vi "Variant_to_string_Core.vi"(11 "Value":variant) -> (3 "1D_Array_String_Setting_Name_Value":string[](array[string]))   [LabVIEW 2011]
uses:
  <vilib>/Utility/VariantDataType/VariantType.lvlib
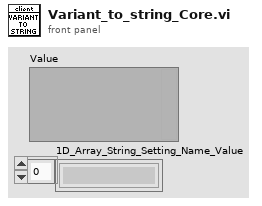
[diagram p1: front panel]
types:
  T1 = typedef "VariantType.lvlib/Type.ctl" = enum8{"Invalid Type", "Void", "I8", "I16", "I32", "I64", "U8", "U16", "U32", "U64", "Single Float", "Double Float", "Extended Float", "Single Complex", "Double Complex", "Extended Complex", "Enum U8", "Enum U16", "Enum U32", "Enum U64", "Single Float With Unit", "Double Float With Unit", "Extended Float With Unit", "Single Complex with Unit", "Double Complex with Unit", "Extended Complex with Unit", "Boolean", "String", "Path", "Picture", "Tag", "Array", "Cluster", "Variant", "LV Variant", "Waveform", "Timestamp", "Digital Waveform", "Digital Data", "ExpressData", "Refnum", "External Data", "VI", "Poly VI", "LabVIEW Class Instance", "Fixed Point"}
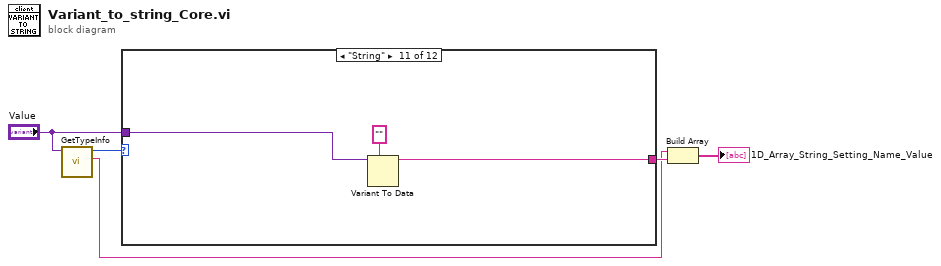
[diagram p0: block diagram]
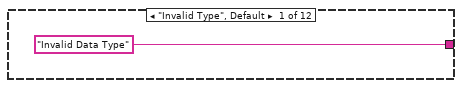
[diagram p2: hidden frame]
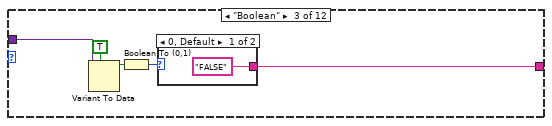
[diagram p4: hidden frame]
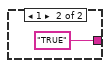
[diagram p5: hidden frame]
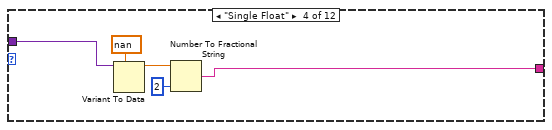
[diagram p6: hidden frame]
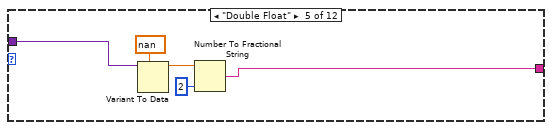
[diagram p7: hidden frame]
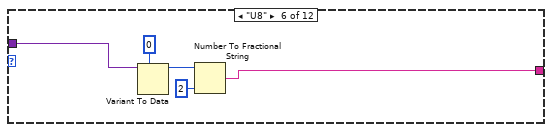
[diagram p8: hidden frame]
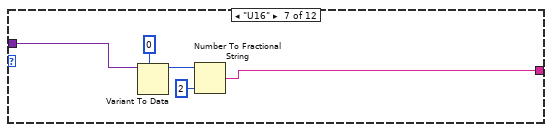
[diagram p9: hidden frame]
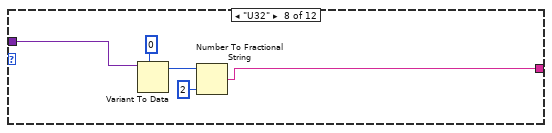
[diagram p10: hidden frame]
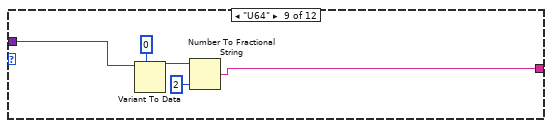
[diagram p11: hidden frame]
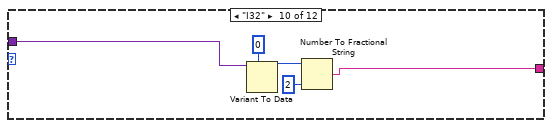
[diagram p12: hidden frame]
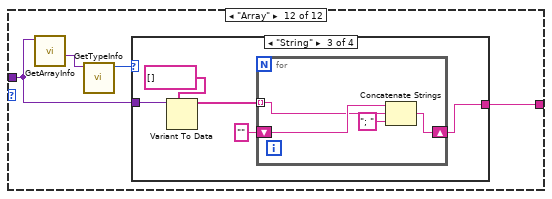
[diagram p13: hidden frame]
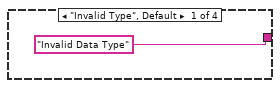
[diagram p14: hidden frame]
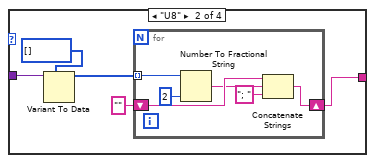
[diagram p15: hidden frame]
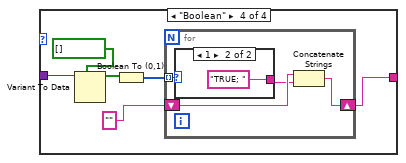
[diagram p16: hidden frame]
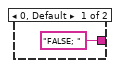
[diagram p17: hidden frame]
diagram:
  n1 = call <vilib>:"GetTypeInfo.vi"("Variant"="Value") -> ("Name"=w2:string, "Type Enum"=w4:T1)  [unwired: 6 in, 3 out]
  n2 = case shown="\"String\"" w4 {
    tunnel: "Value" -> [_ _ w7 w18 w23 w28 w33 w38 w43 w48 w51 w55]
    tunnel: ["Invalid Data Type" _ w10 w15 w20 w25 w30 w34 w39 w44 w49 w52] -> w3
    frame "Invalid Type", Default {
    }
    frame "Enum U16" {
    }
    frame "Boolean" {
      n3 = Variant To Data(type=TRUE, Variant=w7) -> (data=w8:bool)  [unwired: 1 in, 1 out]
      n4 = Boolean To (0,1)(Boolean=w8) -> (0, 1=w11:i16)
      n5 = case shown="0, Default" w11 {
        tunnel: ["FALSE" "TRUE"] -> w10
        frame 0, Default {
        }
        frame 1 {
        }
      }
    }
    frame "Single Float" {
      n6 = Variant To Data(type=sgl nan, Variant=w18) -> (data=w16:sgl)  [unwired: 1 in, 1 out]
      n7 = Number To Fractional String(number=w16, precision (6)=i16 2) -> (F-format string=w15:string)  [unwired: 2 in]
    }
    frame "Double Float" {
      n8 = Variant To Data(type=nan, Variant=w23) -> (data=w21:dbl)  [unwired: 1 in, 1 out]
      n9 = Number To Fractional String(number=w21, precision (6)=i16 2) -> (F-format string=w20:string)  [unwired: 2 in]
    }
    frame "U8" {
      n10 = Variant To Data(type=u8 0, Variant=w28) -> (data=w27:u8)  [unwired: 1 in, 1 out]
      n11 = Number To Fractional String(number=w27, precision (6)=i16 2) -> (F-format string=w25:string)  [unwired: 2 in]
    }
    frame "U16" {
      n12 = Variant To Data(type=u16 0, Variant=w33) -> (data=w32:u16)  [unwired: 1 in, 1 out]
      n13 = Number To Fractional String(number=w32, precision (6)=i16 2) -> (F-format string=w30:string)  [unwired: 2 in]
    }
    frame "U32" {
      n14 = Variant To Data(type=u32 0, Variant=w38) -> (data=w35:u32)  [unwired: 1 in, 1 out]
      n15 = Number To Fractional String(number=w35, precision (6)=i16 2) -> (F-format string=w34:string)  [unwired: 2 in]
    }
    frame "U64" {
      n16 = Variant To Data(type=i16 0, Variant=w43) -> (data=w40:i16)  [unwired: 1 in, 1 out]
      n17 = Number To Fractional String(number=w40, precision (6)=i16 2) -> (F-format string=w39:string)  [unwired: 2 in]
    }
    frame "I32" {
      n18 = Variant To Data(type=0, Variant=w48) -> (data=w45:i32)  [unwired: 1 in, 1 out]
      n19 = Number To Fractional String(number=w45, precision (6)=i16 2) -> (F-format string=w44:string)  [unwired: 2 in]
    }
    frame "String" {
      n20 = Variant To Data(type="", Variant=w51) -> (data=w49:string)  [unwired: 1 in, 1 out]
    }
    frame "Array" {
      n21 = call <vilib>:"GetArrayInfo.vi"("Variant"=w55) -> ("ArrayElement"=w54:variant)  [unwired: 7 in, 3 out]
      n22 = call <vilib>:"GetTypeInfo.vi"("Variant"=w54) -> ("Type Enum"=w53:T1)  [unwired: 6 in, 4 out]
      n23 = case shown="\"String\"" w53 {
        tunnel: ["Invalid Data Type" w58 w69 w77] -> w52
        tunnel: w55 -> [_ w61 w72 w82]
        frame "Invalid Type", Default {
        }
        frame "U8" {
          n24 = Variant To Data(type=u8[] [], Variant=w61) -> (data=w57:u8[])  [unwired: 1 in, 1 out]
          n25 = for {
            shift-right: [w67] -> w58
            shift-left: "" -> [w66]
            tunnel: w57 -> [w64] mode=indexing
            n26 = Number To Fractional String(number=w64, precision (6)=i16 2) -> (F-format string=w63:string)  [unwired: 2 in]
            n27 = Concatenate Strings(w66, w63, "; " ("string")) -> (w67:string)
          }
        }
        frame "String" {
          n28 = Variant To Data(type=string[] [], Variant=w72) -> (data=w68:string[])  [unwired: 1 in, 1 out]
          n29 = for {
            shift-right: [w76] -> w69
            shift-left: "" -> [w75]
            tunnel: w68 -> [w73] mode=indexing
            n30 = Concatenate Strings(w75, w73, "; " ("string")) -> (w76:string)
          }
        }
        frame "Boolean" {
          n31 = Variant To Data(type=bool[] [], Variant=w82) -> (data=w80:bool[])  [unwired: 1 in, 1 out]
          n32 = Boolean To (0,1)(Boolean=w80) -> (0, 1=w79:i16[])
          n33 = for {
            tunnel: w79 -> [w86] mode=indexing
            shift-right: [w85] -> w77
            shift-left: "" -> [w84]
            n34 = case shown="1" w86 {
              tunnel: ["FALSE; " "TRUE; "] -> w83
              frame 0, Default {
              }
              frame 1 {
              }
            }
            n35 = Concatenate Strings(w84, w83) -> (w85:string)
          }
        }
      }
    }
  }
  n36 = Build Array(w2, w3) -> (→"1D_Array_String_Setting_Name_Value":string[])
